vi "Set timer.vi"(6 "Error In":errorcluster, 8 "Target Duration (s)":dbl, 9 "Timer Commands":enum16{"Start timer", "Check timer"}(ring)) -> (0 "Error Out":errorcluster, 2 "Elabsed Time(s)":dbl, 3 "Done?":bool)   [LabVIEW 2019]
panel:
  out "Numeric":dbl
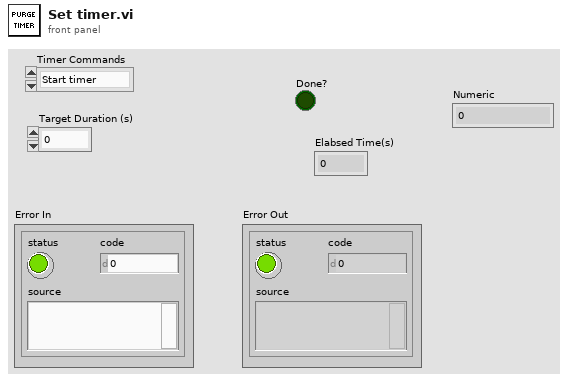
[diagram p1: front panel]
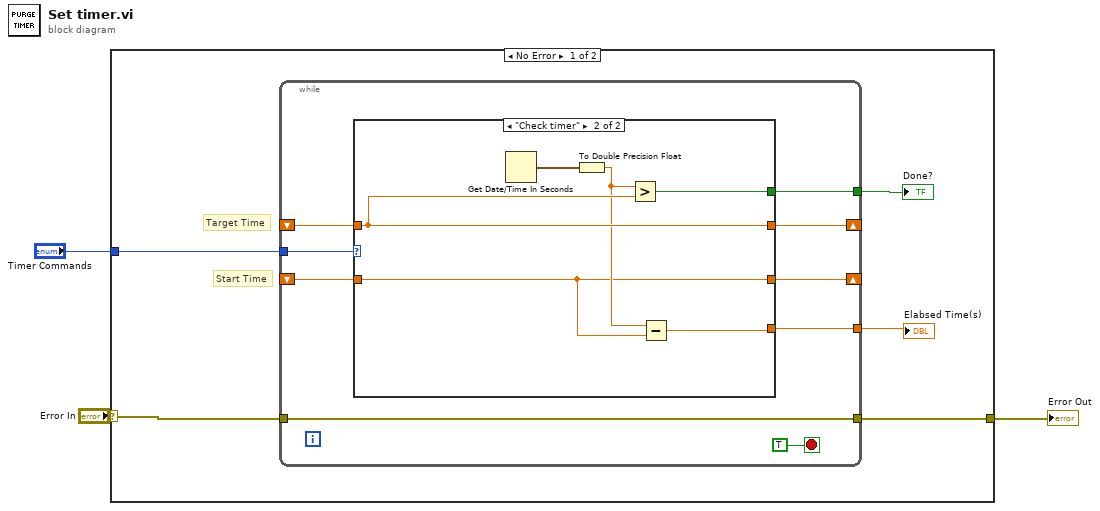
[diagram p0: block diagram]
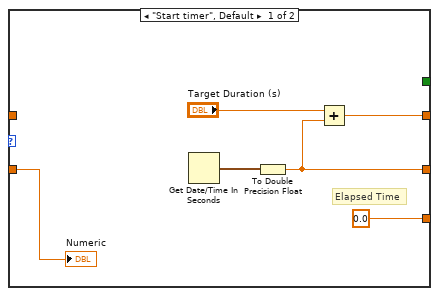
[diagram p2: hidden frame]
diagram:
  n1 = case shown="No Error" "Error In" {
    selector: "Error In" -> [w8 w30]
    tunnel: [w6 w30] -> w2
    tunnel: "Timer Commands" -> [w7 _]
    frame No Error {
      # "Start Time"
      # "Target Time"
      n2 = while {
        tunnel: w8 -> [w10]
        tunnel: w7 -> [w17]
        shift-right: [w16] -> _
        shift-left: _ -> [w15]
        shift-right: [w14] -> _
        shift-left: _ -> [w13]
        tunnel: [w12] -> w5
        tunnel: [w11] -> w4
        tunnel: [w10] -> w6
        stop <- TRUE stop-if-true
        # "Purge process"
        n3 = case shown="\"Check timer\"" w17 {
          tunnel: [w22 w25] -> w16
          tunnel: w15 -> [w18 w25]
          tunnel: [w21 w27] -> w14
          tunnel: w13 -> [_ w27]
          tunnel: [0.0 w24] -> w12
          tunnel: [_ w28] -> w11
          frame "Start timer", Default {
            # "Elapsed Time"
            n4 = Get Date/Time In Seconds() -> (seconds since 1Jan1904=w19:timestamp)
            n5 = To Double Precision Float(number=w19) -> (double precision float=w22:dbl)
            n6 = Add(x="Target Duration (s)", y=w22) -> (x+y=w21:dbl)
            "Numeric" <- w18
          }
          frame "Check timer" {
            n7 = Get Date/Time In Seconds() -> (seconds since 1Jan1904=w29:timestamp)
            n8 = To Double Precision Float(number=w29) -> (double precision float=w26:dbl)
            n9 = Greater?(x=w26, y=w27) -> (0:w28:bool)
            n10 = Subtract(x=w26, y=w25) -> (x-y=w24:dbl)
          }
        }
      }
      "Elabsed Time(s)" <- w5
      "Done?" <- w4
    }
    frame Error {
    }
  }
  "Error Out" <- w2
